vi "Read Roles.vi"(8 "error in (no error)":errorcluster, 11 "TestPlay in":refnum<class "TestPlay.lvclass">) -> (0 "error out":errorcluster, 2 "Roles":T1, 3 "TestPlay out":refnum<class "TestPlay.lvclass">)   [LabVIEW 2023, in "TestPlay.lvclass"]
uses:
  TestPlay.lvclass
  TestRole_class/TestRole.lvclass
  Role_class/Role.lvclass
  SupportAttackerRole/SupportAttackerRole.lvclass
  TestPlay.lvclass/TestPlay.ctl
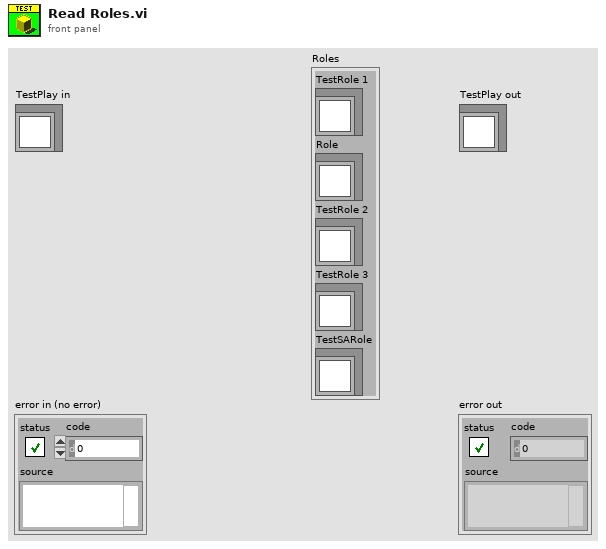
[diagram p1: front panel]
types:
  T1 = cluster{"TestRole 1":refnum<class "TestRole.lvclass">, "Role":refnum<class "Role.lvclass">, "TestRole 2":refnum<class "TestRole.lvclass">, "TestRole 3":refnum<class "TestRole.lvclass">, "TestSARole":refnum<class "SupportAttackerRole.lvclass">}
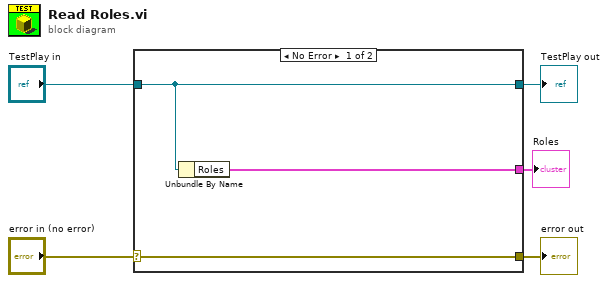
[diagram p0: block diagram]
diagram:
  n1 = case shown="No Error" "error in (no error)" {
    selector: "error in (no error)" -> [w8 w9]
    tunnel: [w8 w9] -> w4
    tunnel: [w7 w10] -> w2
    tunnel: "TestPlay in" -> [w7 w10]
    tunnel: [w6 _] -> w1
    frame No Error {
      n2 = Unbundle By Name(w7) -> ("Roles"=w6:T1)
    }
    frame Error {
    }
  }
  "error out" <- w4
  "TestPlay out" <- w2
  "Roles" <- w1
